vi "InjectPoints.vi"(10 "Distance":dbl=1.0, 11 "Path":cluster{"x":dbl, "y":dbl}[](array[cluster])=[{"x"=80.0, "y"=20.0}, {"x"=260.0, "y"=20.0}, {"x"=260.0, "y"=20.0}]) -> (3 "Path out":cluster{dbl, dbl}[](array[cluster])=[{0.0, 0.0}, {0.9970544855015816, 0.07669649888473705}, {1.9941089710031632, 0.1533929977694741}, {2.991163456504745, 0.23008949665421113}, {3.9882179420063264, 0.3067859955389482}, {4.985272427507908, 0.38348249442368526}, {5.98232691300949, 0.46017899330842227}, {6.979381398511071, 0.5368754921931593}, {7.976435884012653, 0.6135719910778964}, {8.973490369514234, 0.6902684899626335}, {9.970544855015817, 0.7669649888473705}, {10.967599340517397, 0.8436614877321076}, {11.96465382601898, 0.9203579866168445}, {12.96170831152056, 0.9970544855015816}, {13.958762797022143, 1.0737509843863187}, {14.955817282523723, 1.1504474832710558}, {15.952871768025306, 1.2271439821557928}, {16.949926253526886, 1.3038404810405297}, {17.94698073902847, 1.380536979925267}, {18.94403522453005, 1.4572334788100039}, {19.941089710031633, 1.533929977694741}, {20.938144195533212, 1.610626476579478}, {21.935198681034795, 1.6873229754642152}, {22.932253166536377, 1.7640194743489521}, {23.92930765203796, 1.840715973233689}, {24.92636213753954, 1.9174124721184262}, {25.92341662304112, 1.9941089710031632}, {26.920471108542703, 2.0708054698879}, {27.917525594044285, 2.1475019687726373}, {28.914580079545868, 2.2241984676573745}, {29.911634565047446, 2.3008949665421117}, {30.90868905054903, 2.3775914654268484}, {31.90574353605061, 2.4542879643115856}, {32.902798021552194, 2.5309844631963228}, {33.89985250705377, 2.6076809620810595}, {34.89690699255536, 2.6843774609657967}, {35.89396147805694, 2.761073959850534}, {36.891015963558516, 2.837770458735271}, {37.8880704490601, 2.9144669576200077}, {38.88512493456168, 2.991163456504745}, {39.88217942006327, 3.067859955389482}, {40.879233905564845, 3.144556454274219}, {41.876288391066424, 3.221252953158956}, {42.87334287656801, 3.297949452043693}, {43.87039736206959, 3.3746459509284303}, {44.867451847571175, 3.451342449813167}, {45.864506333072754, 3.5280389486979042}, {46.86156081857433, 3.6047354475826414}, {47.85861530407592, 3.681431946467378}, {48.8556697895775, 3.7581284453521153}, {49.85272427507908, 3.8348249442368525}, {50.84977876058066, 3.9115214431215897}, {51.84683324608224, 3.9882179420063264}, {52.84388773158383, 4.064914440891064}, {53.840942217085406, 4.1416109397758}, {54.837996702586985, 4.2183074386605375}, {55.83505118808857, 4.295003937545275}, {56.83210567359015, 4.371700436430012}, {57.829160159091735, 4.448396935314749}, {58.826214644593314, 4.525093434199486}, {59.82326913009489, 4.601789933084223}, {60.82032361559648, 4.67848643196896}, {61.81737810109806, 4.755182930853697}, {62.814432586599644, 4.831879429738434}, {63.81148707210122, 4.908575928623171}, {64.80854155760281, 4.985272427507908}, {65.80559604310439, 5.0619689263926455}, {66.80265052860597, 5.138665425277383}, {67.79970501410754, 5.215361924162119}, {68.79675949960912, 5.292058423046856}, {69.79381398511072, 5.368754921931593}, {70.7908684706123, 5.4454514208163305}, {71.78792295611387, 5.522147919701068}, {72.78497744161545, 5.598844418585805}, {73.78203192711703, 5.675540917470542}, {74.77908641261862, 5.752237416355278}, {75.7761408981202, 5.8289339152400155}, {76.77319538362178, 5.905630414124753}, {77.77024986912336, 5.98232691300949}, {78.76730435462494, 6.059023411894227}, {79.76435884012653, 6.135719910778964}, {80.76141332562811, 6.212416409663701}, {81.75846781112969, 6.289112908548438}, {82.75552229663127, 6.365809407433175}, {83.75257678213285, 6.442505906317912}, {84.74963126763444, 6.519202405202649}, {85.74668575313602, 6.595898904087386}, {86.7437402386376, 6.6725954029721235}, {87.74079472413918, 6.749291901856861}, {88.73784920964076, 6.825988400741597}, {89.73490369514235, 6.902684899626334}, {90.73195818064393, 6.979381398511071}, {91.72901266614551, 7.0560778973958085}, {92.72606715164709, 7.132774396280546}, {93.72312163714867, 7.209470895165283}, {94.72017612265026, 7.28616739405002}, {95.71723060815184, 7.362863892934756}, {96.71428509365342, 7.4395603918194935}, {97.711339579155, 7.516256890704231}, {98.70839406465657, 7.592953389588968}, {99.70544855015817, 7.669649888473705}, {100.70250303565975, 7.746346387358442}, {101.69955752116132, 7.823042886243179}, {102.6966120066629, 7.8997393851279165}, {103.69366649216448, 7.976435884012653}, {104.69072097766607, 8.05313238289739}, {105.68777546316765, 8.129828881782128}, {106.68482994866923, 8.206525380666864}, {107.68188443417081, 8.2832218795516}, {108.67893891967239, 8.359918378436339}, {109.67599340517397, 8.436614877321075}, {110.67304789067556, 8.513311376205813}, {111.67010237617714, 8.59000787509055}, {112.66715686167872, 8.666704373975287}, {113.6642113471803, 8.743400872860024}, {114.66126583268188, 8.82009737174476}, {115.65832031818347, 8.896793870629498}, {116.65537480368505, 8.973490369514234}, {117.65242928918663, 9.050186868398972}, {118.6494837746882, 9.126883367283709}, {119.64653826018979, 9.203579866168447}, {120.64359274569138, 9.280276365053183}, {121.64064723119296, 9.35697286393792}, {122.63770171669454, 9.433669362822657}, {123.63475620219612, 9.510365861707394}, {124.6318106876977, 9.587062360592132}, {125.62886517319929, 9.663758859476868}, {126.62591965870087, 9.740455358361606}, {127.62297414420244, 9.817151857246342}, {128.62002862970402, 9.893848356131079}, {129.61708311520562, 9.970544855015817}, {130.61413760070718, 10.047241353900553}, {131.61119208620877, 10.123937852785291}, {132.60824657171034, 10.200634351670027}, {133.60530105721193, 10.277330850554765}, {134.60235554271352, 10.354027349439502}, {135.5994100282151, 10.430723848324238}, {136.59646451371668, 10.507420347208976}, {137.59351899921825, 10.584116846093712}, {138.59057348471984, 10.66081334497845}, {139.58762797022143, 10.737509843863187}, {140.584682455723, 10.814206342747925}, {141.5817369412246, 10.890902841632661}, {142.57879142672616, 10.967599340517397}, {143.57584591222775, 11.044295839402135}, {144.57290039772934, 11.120992338286872}, {145.5699548832309, 11.19768883717161}, {146.5670093687325, 11.274385336056346}, {147.56406385423406, 11.351081834941084}, {148.56111833973566, 11.42777833382582}, {149.55817282523725, 11.504474832710557}, {150.55522731073881, 11.581171331595295}, {151.5522817962404, 11.657867830480031}, {152.54933628174197, 11.734564329364769}, {153.54639076724357, 11.811260828249505}, {154.54344525274516, 11.887957327134243}, {155.54049973824672, 11.96465382601898}, {156.53755422374832, 12.041350324903716}, {157.53460870924988, 12.118046823788454}, {158.53166319475147, 12.19474332267319}, {159.52871768025307, 12.271439821557928}, {160.52577216575463, 12.348136320442665}, {161.52282665125622, 12.424832819327403}, {162.5198811367578, 12.501529318212139}, {163.51693562225938, 12.578225817096875}, {164.51399010776097, 12.654922315981613}, {165.51104459326254, 12.73161881486635}, {166.50809907876413, 12.808315313751088}, {167.5051535642657, 12.885011812635824}, {168.5022080497673, 12.961708311520562}, {169.49926253526888, 13.038404810405298}, {170.49631702077045, 13.115101309290035}, {171.49337150627204, 13.191797808174773}, {172.4904259917736, 13.268494307059509}, {173.4874804772752, 13.345190805944247}, {174.4845349627768, 13.421887304828983}, {175.48158944827836, 13.498583803713721}, {176.47864393377995, 13.575280302598458}, {177.4756984192815, 13.651976801483194}, {178.4727529047831, 13.728673300367932}, {179.4698073902847, 13.805369799252668}, {180.46686187578626, 13.882066298137406}, {181.46391636128786, 13.958762797022143}, {182.46097084678942, 14.03545929590688}, {183.45802533229102, 14.112155794791617}, {184.4550798177926, 14.188852293676353}, {185.45213430329417, 14.265548792561091}, {186.44918878879577, 14.342245291445828}, {187.44624327429733, 14.418941790330566}, {188.44329775979892, 14.495638289215302}, {189.44035224530052, 14.57233478810004}, {190.43740673080208, 14.649031286984776}, {191.43446121630367, 14.725727785869513}, {192.43151570180524, 14.80242428475425}, {193.42857018730683, 14.879120783638987}, {194.42562467280842, 14.955817282523725}, {195.42267915831, 15.032513781408461}, {196.41973364381158, 15.1092102802932}, {197.41678812931315, 15.185906779177936}, {198.41384261481474, 15.262603278062674}, {199.41089710031633, 15.33929977694741}, {200.4079515858179, 15.415996275832146}, {201.4050060713195, 15.492692774716884}, {202.40206055682106, 15.56938927360162}, {203.39911504232265, 15.646085772486359}, {204.39616952782424, 15.722782271371095}, {205.3932240133258, 15.799478770255833}, {206.3902784988274, 15.87617526914057}, {207.38733298432896, 15.952871768025306}, {208.38438746983056, 16.029568266910044}, {209.38144195533215, 16.10626476579478}, {210.37849644083371, 16.182961264679516}, {211.3755509263353, 16.259657763564256}, {212.37260541183687, 16.336354262448992}, {213.36965989733847, 16.41305076133373}, {214.36671438284003, 16.489747260218465}, {215.36376886834162, 16.5664437591032}, {216.36082335384322, 16.64314025798794}, {217.35787783934478, 16.719836756872677}, {218.35493232484637, 16.796533255757414}, {219.35198681034794, 16.87322975464215}, {220.34904129584953, 16.949926253526886}, {221.34609578135112, 17.026622752411626}, {222.3431502668527, 17.103319251296362}, {223.34020475235428, 17.1800157501811}, {224.33725923785585, 17.256712249065835}, {225.33431372335744, 17.333408747950575}, {226.33136820885903, 17.41010524683531}, {227.3284226943606, 17.486801745720047}, {228.3254771798622, 17.563498244604784}, {229.32253166536375, 17.64019474348952}, {230.31958615086535, 17.71689124237426}, {231.31664063636694, 17.793587741258996}, {232.3136951218685, 17.870284240143732}, {233.3107496073701, 17.94698073902847}, {234.30780409287166, 18.023677237913205}, {235.30485857837326, 18.100373736797945}, {236.30191306387485, 18.17707023568268}, {237.2989675493764, 18.253766734567417}, {238.296022034878, 18.330463233452154}, {239.29307652037957, 18.407159732336893}, {240.29013100588116, 18.48385623122163}, {241.28718549138276, 18.560552730106366}, {242.28423997688432, 18.637249228991102}, {243.28129446238592, 18.71394572787584}, {244.27834894788748, 18.79064222676058}, {245.27540343338907, 18.867338725645315}, {246.27245791889067, 18.94403522453005}, {247.26951240439223, 19.020731723414787}, {248.26656688989382, 19.097428222299524}, {249.2636213753954, 19.174124721184263}, {250.26067586089698, 19.250821220069}, {251.25773034639857, 19.327517718953736}, {252.25478483190014, 19.404214217838472}, {253.25183931740173, 19.480910716723212}, {254.2488938029033, 19.55760721560795}, {255.2459482884049, 19.634303714492685}, {256.2430027739065, 19.71100021337742}, {257.24005725940805, 19.787696712262157}, {258.2371117449096, 19.864393211146897}, {259.23416623041123, 19.941089710031633}, {260.0, 20.0}])   [LabVIEW 2018]
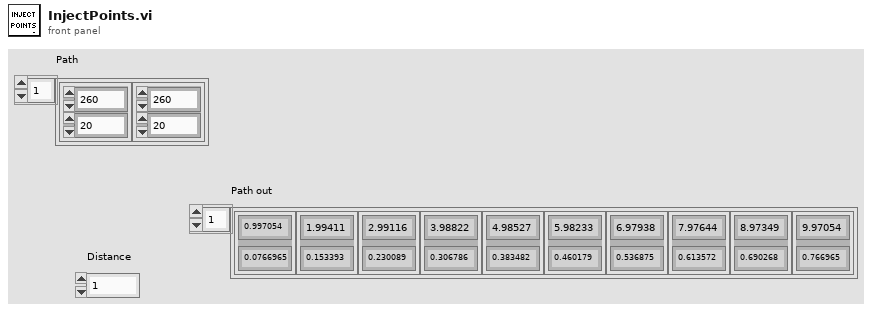
[diagram p1: front panel]
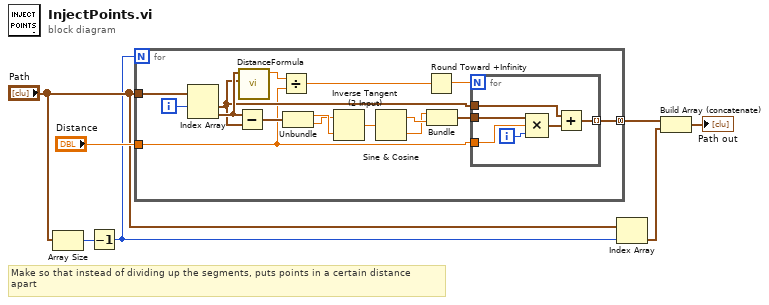
[diagram p0: block diagram]
diagram:
  # "Make so that instead of dividing up the segments, puts points in a certain distance\napart"
  n1 = Array Size(array="Path") -> (size(s)=w7:i32)
  n2 = Decrement(x=w7) -> (x-1=w2:i32)
  n3 = for {
    N: w2 -> [_]
    tunnel: "Path" -> [w23]
    tunnel: "Distance" -> [w12]
    tunnel: [w8] -> w5 mode=concatenating
    i -> [w22]
    n4 = Index Array(array=w23, index #1=w22) -> (element #1=w14:cluster{"x":dbl, "y":dbl}, element #2=w15:cluster{"x":dbl, "y":dbl})  [unwired: 1 in]
    n5 = Subtract(x=w15, y=w14) -> (x-y=w21:cluster{"x":dbl, "y":dbl})
    n6 = call "DistanceFormula.vi"("Point 2"=w14, "Point 1"=w15) -> ("Distance"=w13:dbl)  [unwired: 9 in]
    n7 = Divide(x=w13, y=w12) -> (x/y=w10:dbl)
    n8 = Unbundle(w21) -> ("x"=w20:dbl, "y"=w19:dbl)
    n9 = Inverse Tangent (2 Input)(1:w20, 2:w19) -> (0:w18:dbl)
    n10 = Sine & Cosine(0:w18) -> (1:w17:dbl, 2:w16:dbl)
    n11 = Round Toward +Infinity(x=w10) -> (ceil(x): smallest int >= x=w9:dbl)
    n12 = Bundle(w16, w17) -> (w11:cluster{dbl, dbl})  [unwired: 1 in]
    n13 = for {
      N: w9 -> [_]
      tunnel: w14 -> [w29]
      tunnel: w11 -> [w25]
      tunnel: [w28] -> w8 mode=indexing
      tunnel: w12 -> [w26]
      i -> [w27]
      n14 = Compound Arithmetic op=MULTIPLY(w25, w26, w27) -> (w24:cluster{dbl, dbl})
      n15 = Add(x=w29, y=w24) -> (x+y=w28:cluster{dbl, dbl})
    }
  }
  n16 = Index Array(array="Path", index=w2) -> (element=w1:cluster{"x":dbl, "y":dbl})
  n17 = Build Array (concatenate)(w5, w1) -> (→"Path out":cluster{"x":dbl, "y":dbl}[])
